vi "NI-SWITCH Constants.vi"() -> ()   [LabVIEW 2017, in "NI-SWITCH Scripting.lvlib"]
doc: "Use this Global VI to access the GUIDs assigned to the page resources of the Custom Device."
uses:
  NI-SWITCH Scripting.lvlib
panel:
  in  "Tab Control":T1(tab)=enum."Properties"
  in  "Names.Status":string="Status"
  in  "Names.Endpoint Configuration":string="Endpoint Configuration"
  in  "Properties.Resource":string="Resource"
  in  "Properties.Topology":string="Topology"
  in  "Compiled.Settings":string="Compiled.Settings"
  in  "GUID.SLSC Chassis":string="2d230194-1f79-4241-ad00-e5b0a0d634cb"
  in  "GUID.Status":string="fafe2633-52e8-4be6-bb95-b07e42834d60"
  in  "ChanList.HeartbeatChan":string="Heartbeat"
  in  "ChanList.StatusCode":string="Status code"
  in  "Desc.HeartbeatChan":string="Running count used for debugging. If this channel continues to increment, the custom device is still executing."
  in  "Desc.StatusCode":string="Status code of the custom device. A negative value indicates failure. A positive value indicates warning."
  in  "Paths.CDXML":path=path "SLSC Plugins/Modules/SLSC Switch/SLSC Module SLSC Switch.xml"
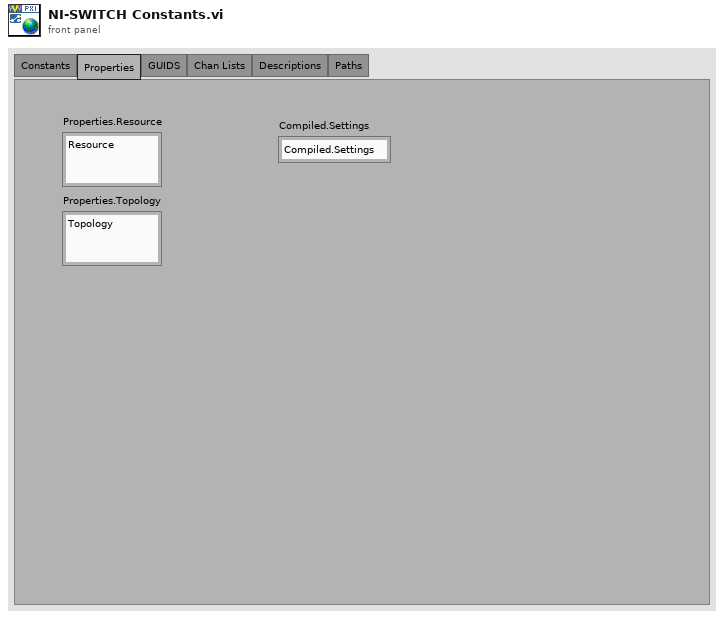
[diagram p1: front panel]
types:
  T1 = enum32{"Constants", "Properties", "GUIDS", "Chan Lists", "Descriptions", "Paths"}
diagram:
